vi "Read from File.vi"(8 "error in (no error)":errorcluster, 10 "INI Ref":T1, 11 "Boolean Assertion in":refnum<class "Boolean Assertion.lvclass">) -> (0 "error out":errorcluster, 2 "INI Ref out":T1, 3 "Boolean Assertion out":refnum<class "Boolean Assertion.lvclass">)   [LabVIEW 2020, in "MacroAssert.lvlib" / "Boolean Assertion.lvclass"]
uses:
  Boolean Assertion.lvclass
  C:/Users/acasalen/Documents/LabVIEW Data/Projects/MacroAssert/source/Classes/Step/Step.lvclass
  <vilib>/Utility/config.llb/Config Data RefNum.ctl
  <vilib>/Utility/config.llb/Read Key (Boolean).vi
  Assertion Step/Assertion Step.lvclass
  <vilib>/Utility/config.llb/NI_LVConfig.lvlib
  MacroAssert.lvlib
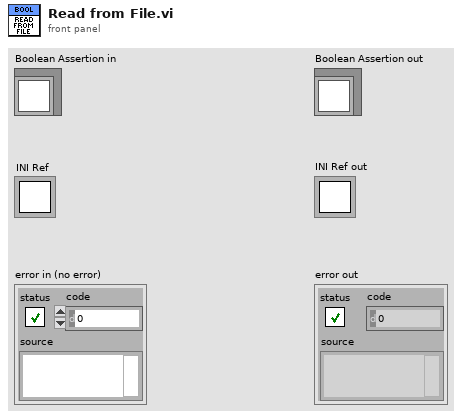
[diagram p1: front panel]
types:
  T1 = typedef "NI_LVConfig.lvlib/Config Data RefNum.ctl" = refnum<k1>
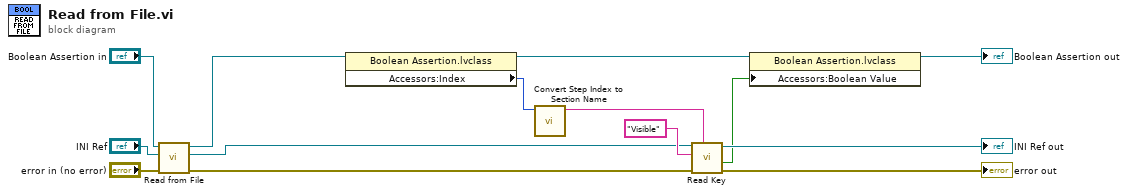
[diagram p0: block diagram]
diagram:
  n1 = call-parent "Read from File.vi"("error in (no error)"="error in (no error)", "INI Ref"="INI Ref", "Assertion Step in"="Boolean Assertion in") -> ("error out"=w4:errorcluster, "INI Ref out"=w1:T1, "Assertion Step out"=w2:refnum<class "Boolean Assertion.lvclass">)  [unwired: 6 in]
  n2 = property class="Boolean Assertion.lvclass"(reference=w2) -> (reference out=w7:refnum<class "Boolean Assertion.lvclass">, "Accessors:Index"=w6:i32)  [unwired: 1 in, 1 out]
  n3 = call "Convert Step Index to Section Name.vi"("Step Index"=w6) -> ("Section Name"=w5:string)  [unwired: 10 in]
  n4 = call-poly <vilib>:"Read Key.vi"("section"=w5, "error in (no error)"=w4, "key"="Visible", "refnum"=w1) -> ("error out"=→"error out":errorcluster, "value"=w8:bool, "refnum out"=→"INI Ref out":T1)  [unwired: 4 in, 1 out]
  n5 = property class="Boolean Assertion.lvclass"(reference=w7, "Accessors:Boolean Value"=w8) -> (reference out=→"Boolean Assertion out":refnum<class "Boolean Assertion.lvclass">)  [unwired: 1 in, 1 out]
